vi "ST5 Goto.vi"(4 "Relatif":bool caption="Relatif/Absolu\n(Absolu)", 5 "error in (no error)":errorcluster, 6 "Mov Ref":refnum<vi>, 7 "Position":dbl caption="Position (mm)" min=-70.0 max=70.0 step=0.0001 format="%#.3g", 8 "Port COM":refnum<visa-resource-name>) -> (0 "error out":errorcluster, 2 "Position Out":dbl caption="Position (mm)" min=0.0 max=119304.64 step=0.018 format="%#.4g", 3 "Port Out":refnum<visa-resource-name>)   [LabVIEW 2010]
doc: "Ce Vi envoie les chaînes de commande au contrôlleur de moteur ST5-Q et vérifie si une réponse se trouve dans le buffer du port série"
uses:
  <userlib>/GenProg/WritebyWeakRefBool.vi
panel:
  in  "Stop":bool caption="En Mouvement"
  out "Réponse":string
  out "Commande":string
  # "Relatif"
  # "Absolu"
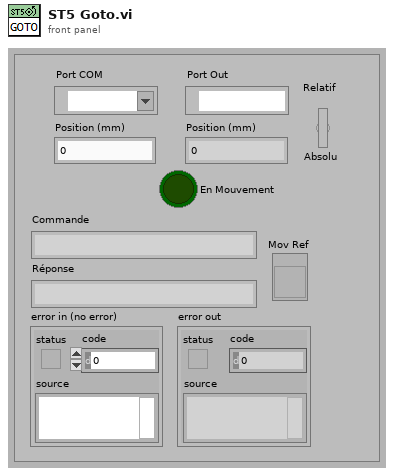
[diagram p1: front panel]
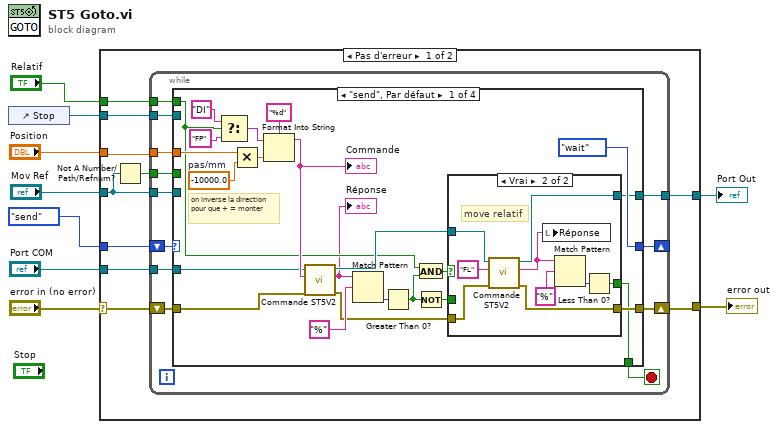
[diagram p0: block diagram]
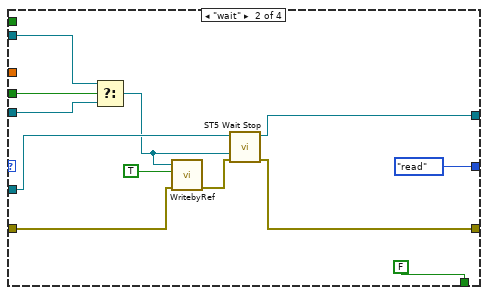
[diagram p3: hidden frame]
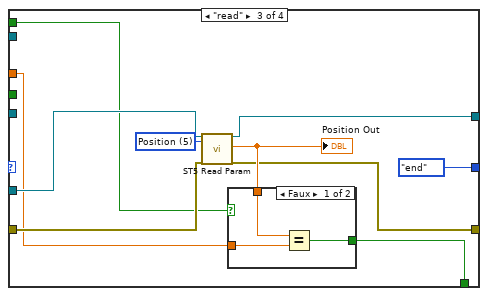
[diagram p4: hidden frame]
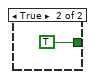
[diagram p5: hidden frame]
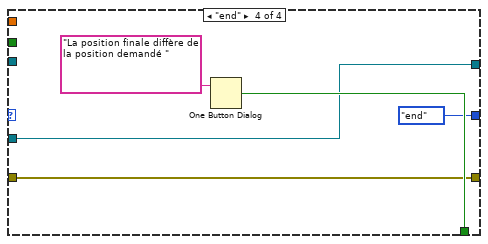
[diagram p6: hidden frame]
diagram:
  n1 = control-ref of="Stop"() -> (w2:refnum<vi>)
  n2 = case shown="Pas d'erreur" "error in (no error)" {
    selector: "error in (no error)" -> [w16 w99]
    tunnel: "Port COM" -> [w17 w98]
    tunnel: [w14 w99] -> w7
    tunnel: "Position" -> [w18 _]
    tunnel: enum16{"send", "wait", "read", "end"}."send" -> [w19 _]
    tunnel: [w15 w98] -> w4
    tunnel: "Mov Ref" -> [w13 _]
    tunnel: w2 -> [w11 _]
    tunnel: "Relatif" -> [w10 _]
    frame No Error {
      n3 = Not A Number/Path/Refnum?(number/path/refnum=w13) -> (NaN/Path/Refnum?=w12:bool)
      n4 = while {
        shift-right: [w24] -> _
        shift-left: w19 -> [w31]
        tunnel: w18 -> [w30]
        tunnel: w17 -> [w29]
        shift-right: [w27] -> w14
        shift-left: w16 -> [w28]
        tunnel: [w26] -> w15
        tunnel: w13 -> [w23]
        tunnel: w12 -> [w22]
        tunnel: w11 -> [w21]
        tunnel: w10 -> [w20]
        stop <- w25 stop-if-true
        n5 = case shown="\"send\", Par défaut" w31 {
          tunnel: w30 -> [w48 _ w83 _]
          tunnel: w29 -> [w47 w78 w87 w94]
          tunnel: w28 -> [w46 w70 w85 w93]
          tunnel: [w40 w77 w80 w93] -> w27
          tunnel: [w39 w76 w86 w94] -> w26
          tunnel: [w38 FALSE w82 w96] -> w25
          tunnel: [enum16{"send", "wait", "read", "end"}."wait" enum16{"send", "wait", "read", "end"}."read" enum16{"send", "wait", "read", "end"}."end" enum16{"send", "wait", "read", "end"}."end"] -> w24
          tunnel: w23 -> [_ w72 _ _]
          tunnel: w22 -> [_ w71 _ _]
          tunnel: w21 -> [_ w73 _ _]
          tunnel: w20 -> [w37 _ w79 _]
          frame "send", Default {
            w49 = -10000.0  # pas/mm
            # "on inverse la direction\npour que + = monter"
            n6 = Select(t="DI" ("chaîne initiale"), s=w37, f="FP" ("chaîne initiale")) -> (s? t:f=w43:string)
            n7 = Multiply(x=w48, y=w49) -> (x*y=w50:dbl)
            n8 = Format Into String(format string="%d" ("chaîne de format"), initial string=w43, w50) -> (resulting string=w52:string)  [unwired: 1 in, 1 out]
            "Commande" <- w52
            n9 = call <userlib>:"Commande ST5V2.vi"("error in (no error)"=w46, "Commande"=w52, "Port COM"=w47) -> ("error out"=w41:errorcluster, "Réponse"=w33:string, "Port Out"=w42:refnum<visa-resource-name>)  [unwired: 2 in]
            "Réponse" <- w33
            n10 = Match Pattern(string=w33, regular expression="%") -> (offset past match=w54:i32)  [unwired: 1 in, 3 out]
            n11 = Greater Than 0?(x=w54) -> (x > 0?=w34:bool)
            n12 = And(x=w37, y=w34) -> (x .and. y?=w35:bool)
            n13 = Not(x=w34) -> (.not. x?=w32:bool)
            n14 = case shown="Vrai" w35 {
              tunnel: w42 -> [w57 w66]
              tunnel: w41 -> [w56 w65]
              tunnel: [w56 w64] -> w40
              tunnel: [w57 w63] -> w39
              tunnel: w32 -> [w55 _]
              tunnel: [w55 w60] -> w38
              frame False {
                # "move absolu"
              }
              frame True {
                # "move relatif"
                n15 = call <userlib>:"Commande ST5V2.vi"("error in (no error)"=w65, "Commande"="FL", "Port COM"=w66) -> ("error out"=w64:errorcluster, "Réponse"=w58:string, "Port Out"=w63:refnum<visa-resource-name>)  [unwired: 2 in]
                n16 = local write "Réponse"(w58) -> ()
                n17 = Match Pattern(string=w58, regular expression="%") -> (offset past match=w61:i32)  [unwired: 1 in, 3 out]
                n18 = Less Than 0?(x=w61) -> (x < 0?=w60:bool)
              }
            }
          }
          frame "wait" {
            n19 = Select(t=w73, s=w71, f=w72) -> (s? t:f=w67:refnum<vi>)
            n20 = call-poly <userlib>:"WritebyRef.vi"("error in"=w70, "Valeur"=TRUE, "Control Ref"=w67) -> ("error out"=w69:errorcluster)  [unwired: 8 in]
            n21 = call <userlib>:"ST5 Wait Stop.vi"("error in"=w69, "Move Ref"=w67, "Port COM"=w78) -> ("error out"=w77:errorcluster, "Port Out"=w76:refnum<visa-resource-name>)  [unwired: 7 in]
          }
          frame "read" {
            w88 = u16 5 items=["All", "Velocity", "Acceleration", "Deceleration", "Max Acceleration", "Position"] ("Parameters")
            n22 = call <userlib>:"ST5 Read Param.vi"("Port COM"=w87, "Parameters"=w88, "error in (no error)"=w85) -> ("Port COM Out"=w86:refnum<visa-resource-name>, "Position"=w84:dbl, "error out"=w80:errorcluster)  [unwired: 10 in, 4 out]
            "Position Out" <- w84
            n23 = case shown="Faux" w79 {
              tunnel: w84 -> [w91 _]
              tunnel: w83 -> [w90 _]
              tunnel: [w89 TRUE] -> w82
              frame False {
                n24 = Equal?(x=w91, y=w90) -> (x = y?=w89:bool)
              }
              frame True {
              }
            }
          }
          frame "end" {
            n25 = One Button Dialog(message="La position finale diffère de la position demandé ") -> (true=w96:bool)  [unwired: 1 in]
          }
        }
      }
    }
    frame Error {
    }
  }
  "error out" <- w7
  "Port Out" <- w4
